vi "BSA_Voltage_Off.vi"(1 "error in":errorcluster) -> (0 "error out":errorcluster)   [LabVIEW 2010]
doc: "The Getting Started Analog Input VI illustrates the basic concepts involved in acquiring analog input data from any data acquisition hardware.\n\nThis VI is explained in detail in the Getting Started with Analog Input section of chapter 1 of the Data Acquisition VI Reference Manual. If you are using SCXI, you should read the Getting Started with SCXI section of chapter 1 first.\n\nAfter you have installed and configured your data acquisition hardware as described in the Installation and Configuration section of chapter 1, you can run this VI to verify your hardware configuration. \n\nYou can pop-up on any front panel object for a description.\n\nIf you are using AMUX-64T boards or SCXI hardware, look at the channels control description for instructions on how to address those external channels; otherwise, you can run the VI with default inputs.\n\nOpen the diagram window to see the data acquisition VI usage."
uses:
  Globals/LDA_meas_global_1.vi
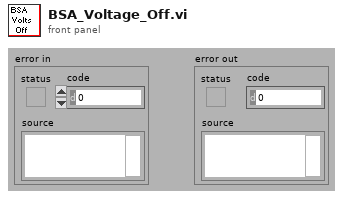
[diagram p1: front panel]
types:
  T1 = typedef "BSA_info_Cluster.ctl" = cluster{"GPIB Address":string, "No of Check Bytes":i32, "Extra Info":string, "COLOUR":u32, "Wavelength (nm)":dbl}
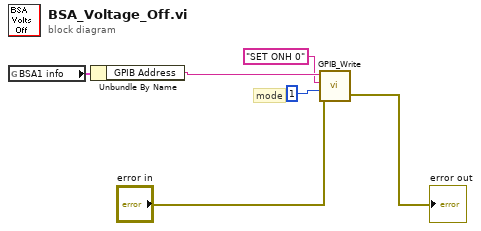
[diagram p0: block diagram]
diagram:
  # "mode"
  n1 = global read "LDA_meas_global_1.vi" "BSA1 info"() -> (w4:T1)
  n2 = Unbundle By Name(w4) -> ("GPIB Address"=w5:string)
  n3 = call "GPIB_Write.vi"("address string"=w5, "data In"="SET ONH 0", "mode (0)"=i16 1, "error in"="error in") -> ("error out"=→"error out":errorcluster)  [unwired: 1 in, 1 out]
